vi "DSF.Engine.Memory.Cache.Framework.Set Plugin Caches.vi"(8 "error in (no error)":errorcluster, 10 "Plugin Caches":refnum<class "DSF.Engine.Memory.Cache.Plugin.lvclass">[](array[class]), 11 "Framework Cache in":refnum<class "DSF.Engine.Memory.Cache.Framework.lvclass">) -> (0 "error out":errorcluster, 3 "Framework Cache out":refnum<class "DSF.Engine.Memory.Cache.Framework.lvclass">)   [LabVIEW 2016, in "DSF.Engine.lvlib" / "DSF.Engine.Memory.Cache.Framework.lvclass"]
uses:
  Cache/DSF.Engine.Memory.Cache.Framework.lvclass
  DSF.Engine.Memory.Cache.Plugin.lvclass
  Cache/DSF.Engine.Memory.Cache.Framework.lvclass/DSF.Engine.Memory.Cache.Framework.ctl
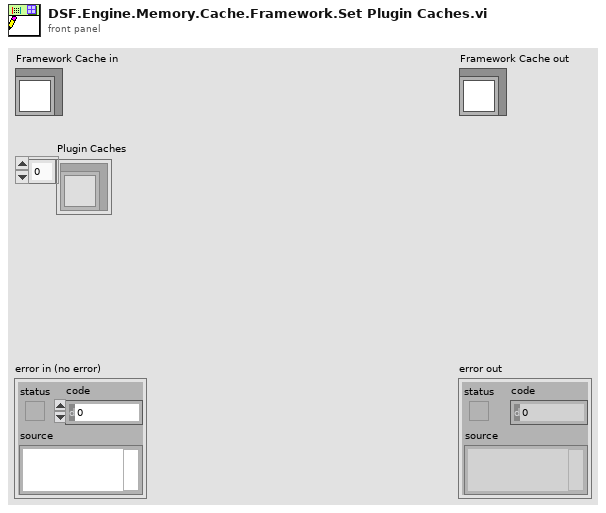
[diagram p1: front panel]
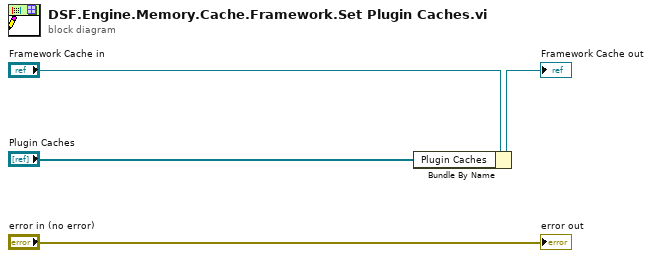
[diagram p0: block diagram]
diagram:
  n1 = Bundle By Name(cluster="Framework Cache in", "Plugin Caches"="Plugin Caches") -> (→"Framework Cache out":refnum<class "DSF.Engine.Memory.Cache.Framework.lvclass">)
  "error out" <- "error in (no error)"
